vi "write measurement requesting hardware devices.vi"(10 "Measurement Name":string, 11 "Respond with Devices for Measurement Msg in":refnum<class "Respond with Devices for Measurement Msg.lvclass">) -> (3 "Respond with Devices for Measurement Msg out":refnum<class "Respond with Devices for Measurement Msg.lvclass">)   [LabVIEW 2016, in "Controller Actor.lvlib" / "Respond with Devices for Measurement Msg.lvclass"]
uses:
  Respond with Devices for Measurement Msg.lvclass
  Respond with Devices for Measurement Msg.lvclass/Respond with Devices for Measurement Msg.ctl
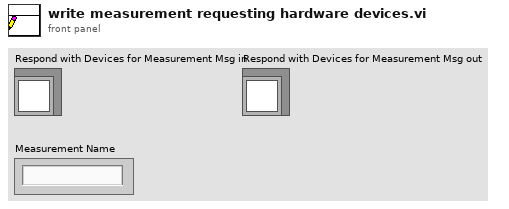
[diagram p1: front panel]
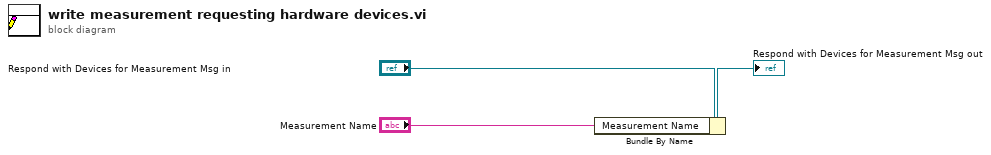
[diagram p0: block diagram]
diagram:
  n1 = Bundle By Name(cluster="Respond with Devices for Measurement Msg in", "Measurement Name"="Measurement Name") -> (→"Respond with Devices for Measurement Msg out":refnum<class "Respond with Devices for Measurement Msg.lvclass">)
